vi "EnterOrExit.vi"(8 "In (T) / Out (F)":bool=TRUE, 9 "Occup array":refnum<vi>[](array[refnum]), 10 "Sense array":refnum<vi>[](array[refnum]), 11 "Occupancy in":T2) -> (3 "Occupancy out":T1)   [LabVIEW 2019]
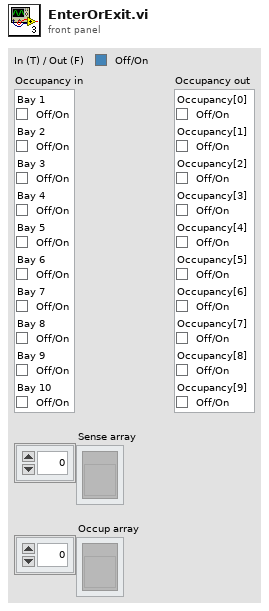
[diagram p1: front panel]
types:
  T1 = cluster{"Occupancy[0]":bool, "Occupancy[1]":bool, "Occupancy[2]":bool, "Occupancy[3]":bool, "Occupancy[4]":bool, "Occupancy[5]":bool, "Occupancy[6]":bool, "Occupancy[7]":bool, "Occupancy[8]":bool, "Occupancy[9]":bool}
  T2 = cluster{"Bay 1":bool, "Bay 2":bool, "Bay 3":bool, "Bay 4":bool, "Bay 5":bool, "Bay 6":bool, "Bay 7":bool, "Bay 8":bool, "Bay 9":bool, "Bay 10":bool}
  T3 = cluster{"Occupancy in[0]":bool, "Occupancy in[1]":bool, "Occupancy in[2]":bool, "Occupancy in[3]":bool, "Occupancy in[4]":bool, "Occupancy in[5]":bool, "Occupancy in[6]":bool, "Occupancy in[7]":bool, "Occupancy in[8]":bool, "Occupancy in[9]":bool}
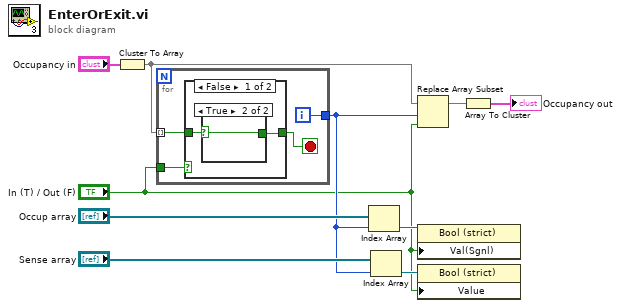
[diagram p0: block diagram]
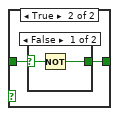
[diagram p3: hidden frame]
diagram:
  n1 = Cluster To Array(cluster="Occupancy in") -> (array=w9:bool[])
  n2 = for {
    tunnel: w9 -> [w14] mode=indexing
    tunnel: [w12] -> w3
    tunnel: "In (T) / Out (F)" -> [w11]
    i -> [w12]
    stop <- w13 stop-if-true
    n3 = case shown="False" w11 {
      tunnel: w14 -> [w16 w19]
      tunnel: [w15 w18] -> w13
      frame False {
        n4 = case shown="True" w16 {
          selector: w16 -> [_ w17]
          tunnel: [_ w17] -> w15
          frame False {
          }
          frame True {
          }
        }
      }
      frame True {
        n5 = case shown="False" w19 {
          selector: w19 -> [w21 _]
          tunnel: [w20 _] -> w18
          frame False {
            n6 = Not(x=w21) -> (.not. x?=w20:bool)
          }
          frame True {
          }
        }
      }
    }
  }
  n7 = Index Array(array="Occup array", index=w3) -> (element=w5:refnum<vi>)
  n8 = Index Array(array="Sense array", index=w3) -> (element=w2:refnum<vi>)
  n9 = Replace Array Subset(array=w9, new element="In (T) / Out (F)", index=w3) -> (w7:bool[])
  n10 = property class="Bool (strict)"(reference=w5, "Val(Sgnl)"="In (T) / Out (F)") -> ()  [unwired: 1 in, 2 out]
  n11 = property class="Bool (strict)"(reference=w2, "Value"="In (T) / Out (F)") -> ()  [unwired: 1 in, 2 out]
  n12 = Array To Cluster(array=w7) -> (cluster=→"Occupancy out":T3)
